vi "Syringe State.vi"(7 "Get/Set":enum16{"Get", "Set"}(ring), 8 "error in (no error)":errorcluster, 9 "Syringe in":T1, 11 "FlexWorktable in":refnum<class "FlexWorktable.lvclass">) -> (0 "error out":errorcluster, 1 "Syringe out":T1, 3 "FlexWorktable out":refnum<class "FlexWorktable.lvclass">)   [LabVIEW 2024, in "FlexWorktable.lvclass"]
uses:
  FlexWorktable.lvclass
  Vec3d Class/Vec3d.lvclass
panel:
  # "Syringe Holder States:\n  - Empty\n  - Populated\n  - Calibrated"
  # "Syringe Holder States:\n  - Empty\n  - Populated\n  - Calibrated"
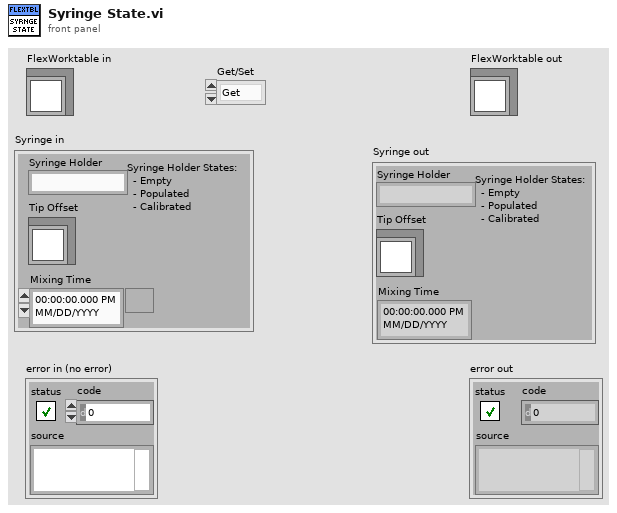
[diagram p1: front panel]
types:
  T1 = cluster{"Syringe Holder":string, "Mixing Time":timestamp, "Tip Offset":refnum<class "Vec3d.lvclass">}
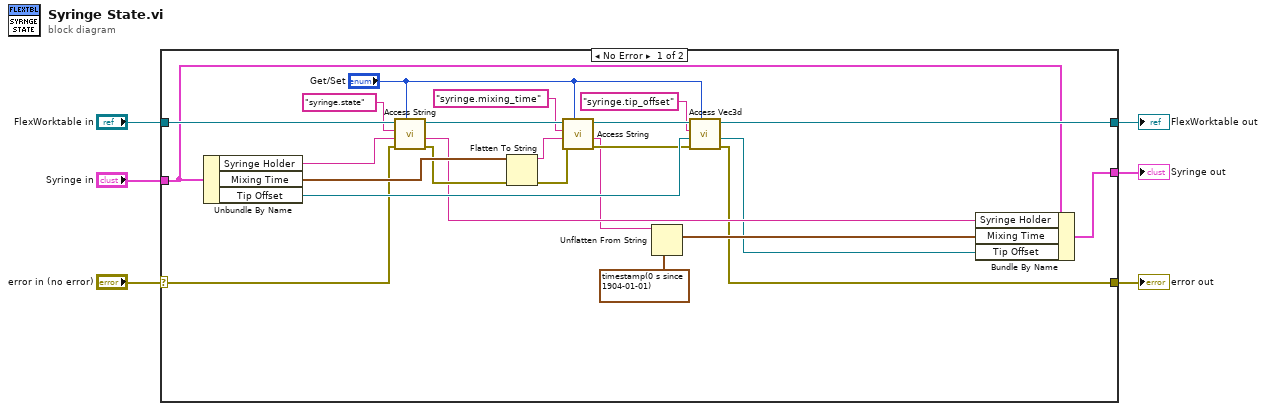
[diagram p0: block diagram]
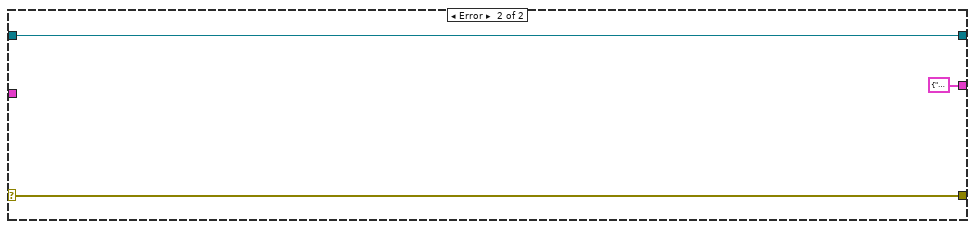
[diagram p2: hidden frame]
diagram:
  n1 = case shown="No Error" "error in (no error)" {
    selector: "error in (no error)" -> [w22 w33]
    tunnel: [w8 w33] -> w5
    tunnel: [w15 w32] -> w3
    tunnel: "FlexWorktable in" -> [w29 w32]
    tunnel: "Syringe in" -> [w14 _]
    tunnel: [w7 T1 {"Syringe Holder"="", "Mixing Time"=timestamp(0 s since 1904-01-01), "Tip Offset"=refnum} ("Syringe in")] -> w1
    frame No Error {
      n2 = Unbundle By Name(w14) -> ("Syringe Holder"=w26:string, "Mixing Time"=w30:timestamp, "Tip Offset"=w23:refnum<class "Vec3d.lvclass">)
      n3 = call-dynamic "Access String.vi"("Get/Set"="Get/Set", "error in (no error)"=w22, "Value in"=w26, "Key"="syringe.state", "FlexWorktable in"=w29) -> ("error out"=w21:errorcluster, "Value out"=w12:string, "FlexWorktable out"=w28:refnum<class "FlexWorktable.lvclass">)  [unwired: 4 in]
      n4 = Flatten To String(anything=w30, error in (no error)=w21) -> (data string=w24:string, error out=w20:errorcluster)  [unwired: 2 in, 1 out]
      n5 = call-dynamic "Access String.vi"("Get/Set"="Get/Set", "error in (no error)"=w20, "Value in"=w24, "Key"="syringe.mixing_time", "FlexWorktable in"=w28) -> ("error out"=w19:errorcluster, "Value out"=w11:string, "FlexWorktable out"=w27:refnum<class "FlexWorktable.lvclass">)  [unwired: 4 in]
      n6 = Unflatten From String(type=timestamp(0 s since 1904-01-01) ("Mixing Time"), binary string=w11) -> (value=w10:timestamp)  [unwired: 3 in, 2 out]
      n7 = call-dynamic "Access Vec3d.vi"("Get/Set"="Get/Set", "error in (no error)"=w19, "Value in"=w23, "Key"="syringe.tip_offset", "FlexWorktable in"=w27) -> ("error out"=w8:errorcluster, "Value out"=w9:refnum<class "Vec3d.lvclass">, "FlexWorktable out"=w15:refnum<class "FlexWorktable.lvclass">)  [unwired: 4 in]
      n8 = Bundle By Name(cluster=w14, "Syringe Holder"=w12, "Mixing Time"=w10, "Tip Offset"=w9) -> (w7:T1)
    }
    frame Error {
    }
  }
  "error out" <- w5
  "FlexWorktable out" <- w3
  "Syringe out" <- w1
